vi "molecularProperties.vi"(11 "Gas":T1) -> (1 "VdWb(L/mol)":dbl, 2 "VdWa(L^2bar/mol^2)":dbl, 3 "Molecular Weight":dbl)   [LabVIEW 2021]
uses:
  Anemometry/Anemometry Sub Vis/Controls/GasCombo.ctl
panel:
  # "https://en.wikipedia.org/wiki/Van_der_Waals_constants_(data_page)"
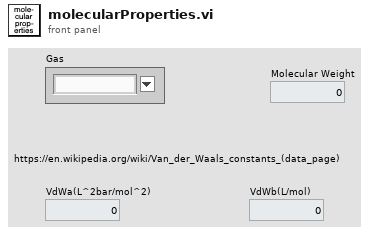
[diagram p1: front panel]
types:
  T1 = typedef "GasCombo.ctl" = string
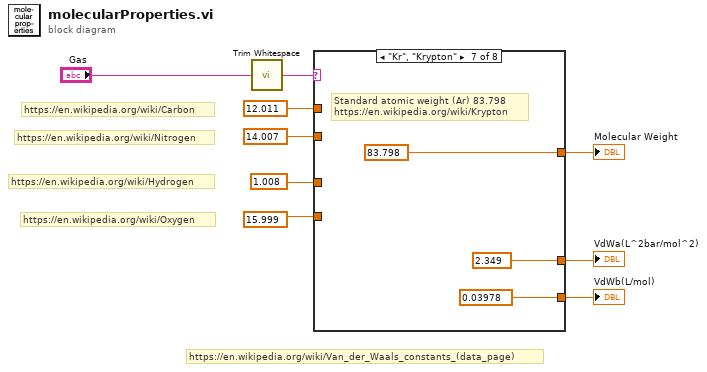
[diagram p0: block diagram]
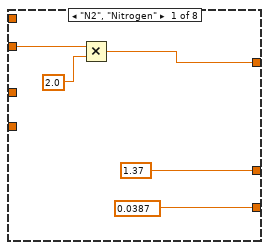
[diagram p2: hidden frame]
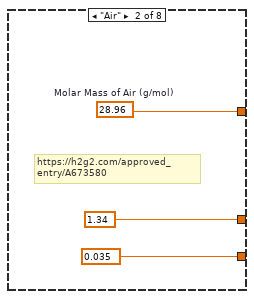
[diagram p3: hidden frame]
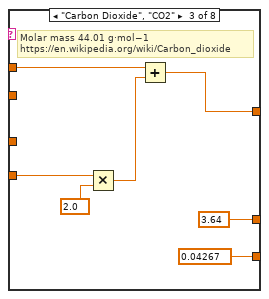
[diagram p4: hidden frame]
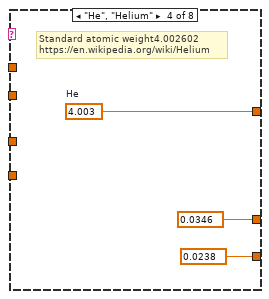
[diagram p5: hidden frame]
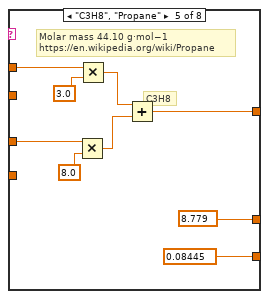
[diagram p6: hidden frame]
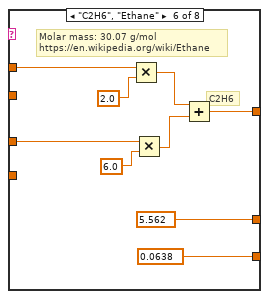
[diagram p7: hidden frame]
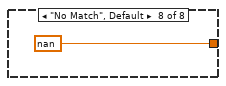
[diagram p8: hidden frame]
diagram:
  # "https://en.wikipedia.org/wiki/Van_der_Waals_constants_(data_page)"
  # "https://en.wikipedia.org/wiki/Nitrogen"
  # "https://en.wikipedia.org/wiki/Oxygen"
  # "https://en.wikipedia.org/wiki/Hydrogen"
  # "https://en.wikipedia.org/wiki/Carbon"
  n1 = call <vilib>:"Trim Whitespace.vi"("string"="Gas") -> ("trimmed string"=w2:string)  [unwired: 1 in]
  n2 = case shown="\"Kr\", \"Krypton\"" w2 {
    tunnel: [w13 w17 w22 w27 w32 w41 83.798 nan] -> w1
    tunnel: 12.011 ("C") -> [_ _ w21 _ w31 w40 _ _]
    tunnel: 1.008 ("H") -> [_ _ _ _ w30 w39 _ _]
    tunnel: 15.999 ("O") -> [_ _ w20 _ _ _ _ _]
    tunnel: 14.007 ("N") -> [w12 _ _ _ _ _ _ _]
    tunnel: [1.37 1.34 3.64 ("VdWa(L^2mBar/mol^2)") 0.0346 ("VdWa(L^2mBar/mol^2)") 8.779 5.562 2.349 ("VdWa(L^2mBar/mol^2)") _] -> w8
    tunnel: [0.0387 0.035 0.04267 ("VdWb(L/mol)") 0.0238 ("VdWb(L/mol)") 0.08445 0.0638 0.03978 ("VdWb(L/mol)") _] -> w9
    frame "N2", "Nitrogen" {
      n3 = Multiply(x=w12, y=2.0) -> (x*y=w13:dbl)
    }
    frame "Air" {
      w17 = 28.96  # Molar Mass of Air (g/mol)
      # "https://h2g2.com/approved_entry/A673580"
    }
    frame "Carbon Dioxide", "CO2" {
      # "Molar mass\t44.01 g·mol−1\nhttps://en.wikipedia.org/wiki/Carbon_dioxide"
      n4 = Multiply(x=w20, y=2.0 ("O")) -> (x*y=w24:dbl)
      n5 = Add(x=w21, y=w24) -> (x+y=w22:dbl)
    }
    frame "He", "Helium" {
      w27 = 4.003  # He
      # "Standard atomic weight4.002602\nhttps://en.wikipedia.org/wiki/Helium"
    }
    frame "C3H8", "Propane" {
      # "Molar mass\t44.10 g·mol−1\nhttps://en.wikipedia.org/wiki/Propane"
      # "C3H8"
      n6 = Multiply(x=w30, y=8.0) -> (x*y=w33:dbl)
      n7 = Multiply(x=w31, y=3.0) -> (x*y=w34:dbl)
      n8 = Add(x=w34, y=w33) -> (x+y=w32:dbl)
    }
    frame "C2H6", "Ethane" {
      # "Molar mass: 30.07 g/mol\nhttps://en.wikipedia.org/wiki/Ethane"
      # "C2H6"
      n9 = Multiply(x=w40, y=2.0) -> (x*y=w43:dbl)
      n10 = Multiply(x=w39, y=6.0) -> (x*y=w42:dbl)
      n11 = Add(x=w43, y=w42) -> (x+y=w41:dbl)
    }
    frame "Kr", "Krypton" {
      # "Standard atomic weight (Ar)\t83.798\nhttps://en.wikipedia.org/wiki/Krypton"
    }
    frame "No Match", Default {
    }
  }
  "VdWb(L/mol)" <- w9
  "VdWa(L^2bar/mol^2)" <- w8
  "Molecular Weight" <- w1
